vi "Generate Digital Pulse.vi"   [LabVIEW 2017, in "NI_Robotics_FPGA Utilities.lvlib"]
uses:
  <vilib>/robotics/Utilities/FPGA Utilities/NI_Robotics_FPGA Utilities.lvlib
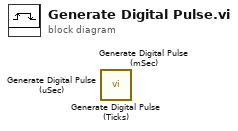
[diagram p0: block diagram]
diagram:
  n1 = call <vilib>:"Generate Digital Pulse (Ticks).vi"() -> ()  [unwired: 12 in]
  n2 = call <vilib>:"Generate Digital Pulse (mSec).vi"() -> ()  [unwired: 12 in]
  n3 = call <vilib>:"Generate Digital Pulse (uSec).vi"() -> ()  [unwired: 12 in]
